vi "Main Action Process Ctrl.vi"(7 "Action":T2(ring)=enum."Delete & Check", 8 "error in":errorcluster, 9 "index":i32, 10 "Add Action Que":T1[](array[typedef])) -> (0 "Finish":bool, 1 "Delete Action":T1, 2 "Count":i32, 3 "Read Action":T1)   [LabVIEW 2019]
uses:
  Ctrl/Process Action Name.ctl
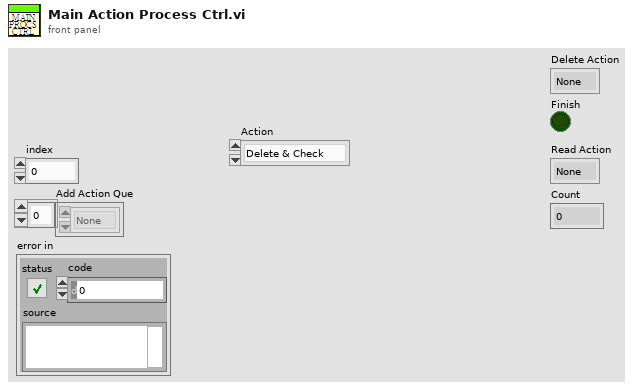
[diagram p1: front panel]
types:
  T1 = typedef "Process Action Name.ctl" = enum16{"None", "*******Initial*******", "*******Check Run*******", "*******Manual*******", "*******Others*******", "*******Exit*******", "Exit"}
  T2 = enum16{"Initial", "Add", "Read", "Delete & Check"}
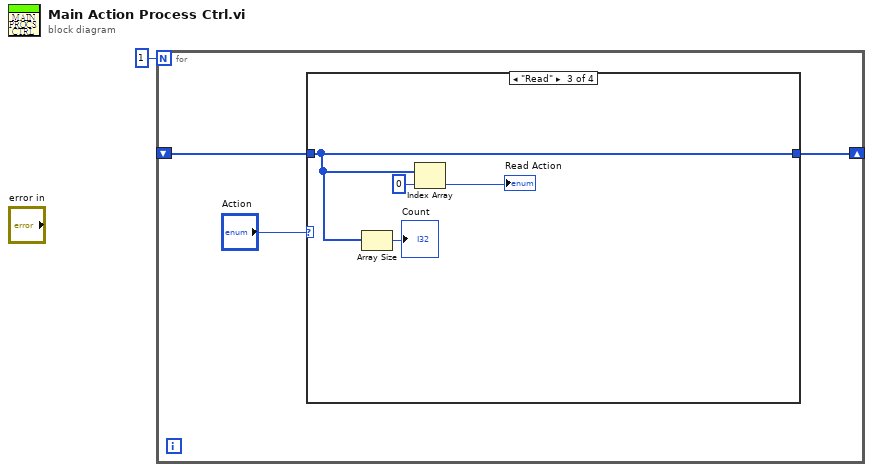
[diagram p0: block diagram]
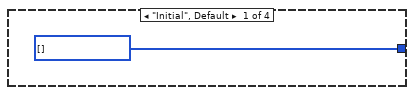
[diagram p2: hidden frame]
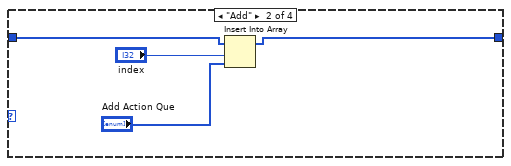
[diagram p3: hidden frame]
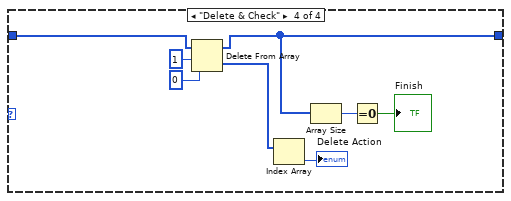
[diagram p4: hidden frame]
diagram:
  n1 = for {
    N: 1 -> [_]
    shift-right: [w4] -> _
    shift-left: _ -> [w3]
    n2 = case shown="\"Read\"" "Action" {
      tunnel: [w5 w8 w11 w20] -> w4
      tunnel: w3 -> [_ w9 w11 w21]
      frame "Initial", Default {
        w5 = T1[] [] items=["None", "*******Initial*******", "*******Check Run*******", "*******Manual*******", "*******Others*******", "*******Exit*******", "Exit"]
      }
      frame "Add" {
        n3 = Insert Into Array(array=w9, index="index", new element="Add Action Que") -> (w8:T1[])
      }
      frame "Read" {
        n4 = Array Size(array=w11) -> (size(s)=→"Count":i32)
        n5 = Index Array(array=w11, index=0) -> (element=→"Read Action":T1)
      }
      frame "Delete & Check" {
        n6 = Delete From Array(array=w21, length=1, index=0) -> (deleted portion=w17:T1[], array with subset deleted=w20:T1[])
        n7 = Index Array(array=w17) -> (element=→"Delete Action":T1)  [unwired: 1 in]
        n8 = Array Size(array=w20) -> (size(s)=w15:i32)
        n9 = Equal To 0?(x=w15) -> (x = 0?=→"Finish":bool)
      }
    }
  }
